vi "DHE_GetElapsedExpTime.vi"() -> (2 "ElapsedExp":u32)   [LabVIEW 2016]
uses:
  private/vis/DHE_VarAction.ctl
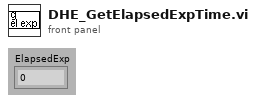
[diagram p1: front panel]
types:
  T1 = typedef "DHE_VarAction.ctl" = enum16{"read", "write"}
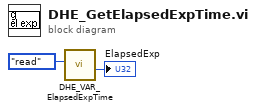
[diagram p0: block diagram]
diagram:
  n1 = call "DHE_VAR_ElapsedExpTime.vi"("action"=DHE_VarAction."read") -> ("ElapsedExp"=→"ElapsedExp":u32)  [unwired: 1 in, 9 out]
